vi "Calculate Particle Scores_Custom.vi"(7 "Pixel Value":i32=1, 8 "Limit Tests?":bool=TRUE, 9 "Aspect Fudge Factor":dbl=1.0, 10 "Sorted Data":dbl[][](array[numeric]), 11 "Image in":T2) -> (3 "Scores":T1[](array[typedef]))   [LabVIEW 2015]
doc: "Calculate scores based on the particle measurements. Calculated scores are for aspect ratio, area to convex hull area, masking, and moment of inertia. These scores range between 0 and 100 and can be used to categorize particles as targets and non-targets. The fudge factor compensates for camera modes that do not give square pixels."
uses:
  <vilib>/vision/Image Controls.llb/IMAQ Image.ctl
  Scores.ctl
  <vilib>/vision/NI_Vision_Development_Module.lvlib
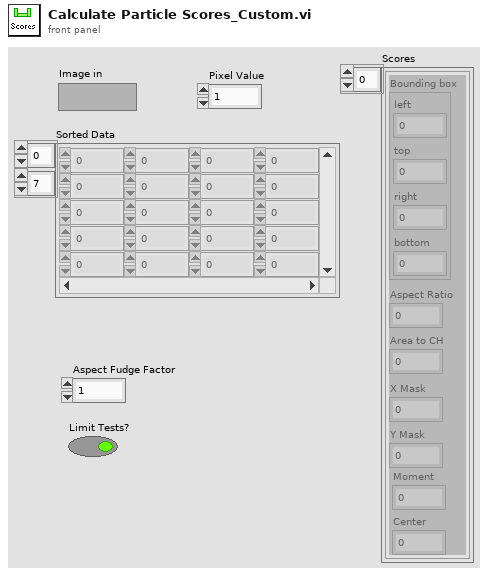
[diagram p1: front panel]
types:
  T1 = typedef "Scores.ctl" = cluster{"Bounding box":cluster{"left":dbl, "top":dbl, "right":dbl, "bottom":dbl}, "Aspect Ratio":dbl, "Area to CH":dbl, "X Mask":dbl, "Y Mask":dbl, "Moment":dbl, "Center":dbl}
  T2 = typedef "IMAQ Image.ctl" = refnum<image>
  T3 = cluster{"[0]":dbl, "[1]":dbl, "[2]":dbl, "[3]":dbl}
  T4 = cluster{cluster{"[0]":dbl, "[1]":dbl, "[2]":dbl, "[3]":dbl}, "Aspect Ratio Score":dbl, "Score":dbl, "X Score":dbl, "Y Score":dbl, "Score":dbl, dbl}
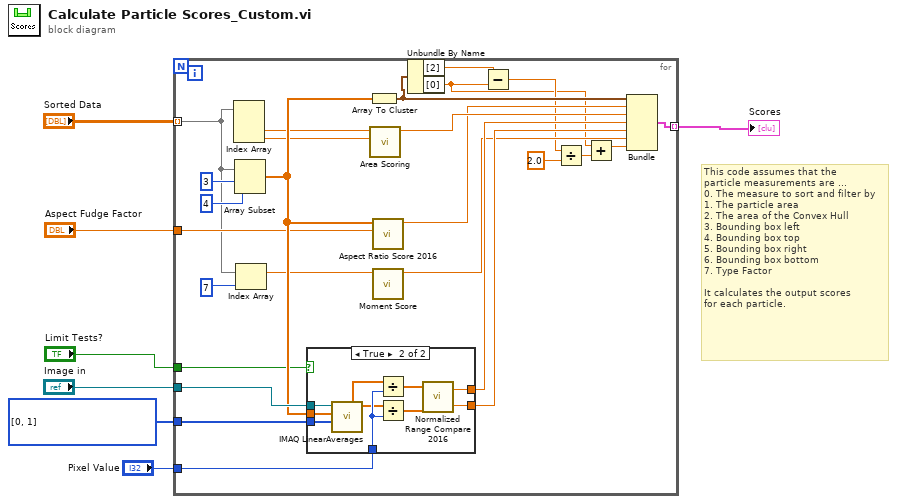
[diagram p0: block diagram]
diagram:
  w5 = i32[] [0, 1] items=["X Axis Averages", "Y Axis Averages", "X + Y Axis Averages", "X - Y Axis Averages"] ("Averages")
  # "This code assumes that the\nparticle measurements are ...\n0. The measure to sort and filter by\n1. The particle area\n2. The area of the Convex Hull\n3. Bounding box left\n4. Bounding box top\n5. Bounding box right\n6. Bounding box bottom\n7. Type Factor\n\nIt calculates the output scores\nfor each particle."
  n1 = for {
    tunnel: "Image in" -> [w29]
    tunnel: "Sorted Data" -> [w18] mode=indexing
    tunnel: [w31] -> w6 mode=indexing
    tunnel: w5 -> [w25]
    tunnel: "Pixel Value" -> [w23]
    tunnel: "Aspect Fudge Factor" -> [w20]
    tunnel: "Limit Tests?" -> [w19]
    n2 = Index Array(array=w18) -> (element #2=w22:dbl, element #3=w21:dbl)  [unwired: 3 in, 1 out]
    n3 = Array Subset(array=w18, index=3, length=4) -> (w24:dbl[])
    n4 = Index Array(array=w18, index=7 ("length")) -> (element=w16:dbl)
    n5 = case shown="True" w19 {
      tunnel: w29 -> [_ w43]
      tunnel: [_ w42] -> w27
      tunnel: [_ w41] -> w26
      tunnel: w25 -> [_ w40]
      tunnel: w24 -> [_ w39]
      tunnel: w23 -> [_ w38]
      frame False {
      }
      frame True {
        n6 = call "IMAQ LinearAverages"("Averages"=w40, "Optional Rectangle"=w39, "Image Src"=w43) -> ("Y Axis Averages"=w36:sgl[], "X Axis Averages"=w37:sgl[])  [unwired: 4 in, 3 out]
        n7 = Divide(x=w37, y=w38) -> (x/y=w35:sgl[])
        n8 = Divide(x=w36, y=w38) -> (x/y=w34:sgl[])
        n9 = call "Normalized Range Compare 2016.vi"("Y Averages"=w34, "X Averages"=w35) -> ("Y Score"=w41:dbl, "X Score"=w42:dbl)
      }
    }
    n10 = Array To Cluster(array=w24) -> (cluster=w14:T3)
    n11 = call "Area Scoring.vi"("Convex Hull Area"=w21, "Area"=w22) -> ("Score"=w30:dbl)  [unwired: 9 in]
    n12 = call "Aspect Ratio Score 2016.vi"("Aspect Fudge Factor"=w20, "Rectangle Array ltrb"=w24) -> ("Aspect Ratio Score"=w28:dbl)  [unwired: 9 in]
    n13 = call "Moment Score.vi"("Moment Factor"=w16) -> ("Score"=w15:dbl)  [unwired: 10 in]
    n14 = Unbundle By Name(w14) -> ("[2]"=w13:dbl, "[0]"=w9:dbl)
    n15 = Subtract(x=w13, y=w9) -> (x-y=w11:dbl)
    n16 = Divide(x=w11, y=2.0) -> (x/y=w8:dbl)
    n17 = Add(x=w9, y=w8) -> (x+y=w12:dbl)
    n18 = Bundle(w14, "Aspect Ratio Score"=w28, "Score"=w30, "X Score"=w27, "Y Score"=w26, "Score"=w15, w12) -> (w31:T4)  [unwired: 1 in]
  }
  "Scores" <- w6
